vi "Save Data（Feedback）.vi"(6 "index":i32, 7 "Data":variant, 8 "error in (no error)":errorcluster caption="错误输入（无错误）", 9 "Code":string, 10 "Table":string, 11 "Connncet State":T1) -> (0 "error out":errorcluster caption="错误输出", 2 "State":bool)   [LabVIEW 2014]
uses:
  <vilib>/addons/database/NI_Database_API.lvlib
  Ctr/Constr.ctl
  <vilib>/addons/database/Connection.llb/Conn ObjectReference.ctl
  Ctr/Conneect State.ctl
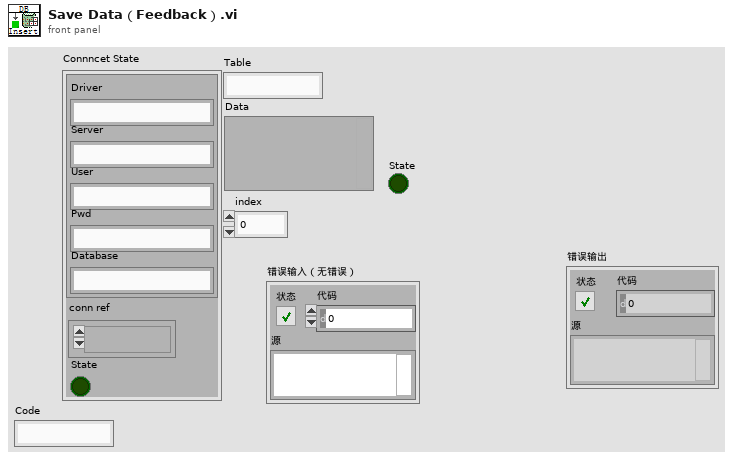
[diagram p1: front panel]
types:
  T1 = typedef "Conneect State.ctl" = cluster{"Constr":T2, "conn ref":T3, "State":bool}
  T2 = typedef "Constr.ctl" = cluster{"Driver":string, "Server":string, "User":string, "Pwd":string, "Database":string}
  T3 = typedef "NI_Database_API.lvlib/Conn ObjectReference.ctl" = refnum<k1>
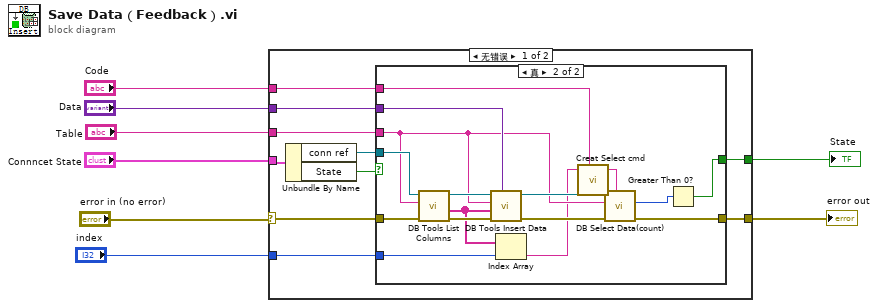
[diagram p0: block diagram]
diagram:
  n1 = case shown="无错误" "error in (no error)" {
    selector: "error in (no error)" -> [w16 w36]
    tunnel: "Connncet State" -> [w18 _]
    tunnel: "Table" -> [w14 _]
    tunnel: "Data" -> [w13 _]
    tunnel: "index" -> [w12 _]
    tunnel: "Code" -> [w11 _]
    tunnel: [w10 w36] -> w2
    tunnel: [w9 _] -> w1
    frame No Error {
      n2 = Unbundle By Name(w18) -> ("conn ref"=w15:T3, "State"=w17:bool)
      n3 = case shown="真" w17 {
        tunnel: w16 -> [w19 w35]
        tunnel: w15 -> [_ w34]
        tunnel: w14 -> [_ w26]
        tunnel: w13 -> [_ w31]
        tunnel: w12 -> [_ w29]
        tunnel: w11 -> [_ w24]
        tunnel: [w19 w23] -> w10
        tunnel: [_ w21] -> w9
        frame False {
        }
        frame True {
          n4 = call <vilib>:"DB Tools List Columns.vi"("error in (no error)"=w35, "table"=w26, "connection reference"=w34) -> ("error out"=w33:errorcluster, "columns"=w30:string[], "connection reference out"=w32:T3)  [unwired: 1 in, 1 out]
          n5 = call <vilib>:"DB Tools Insert Data.vi"("data"=w31, "error in (no error)"=w33, "columns"=w30, "table"=w26, "connection reference"=w32) -> ("error out"=w28:errorcluster, "connection reference out"=w27:T3)  [unwired: 5 in]
          n6 = Index Array(array=w30, index=w29) -> (element=w25:string)
          n7 = call "Creat Select cmd.vi"("Col"=w25, "Code"=w24) -> ("Str"=w20:string)  [unwired: 7 in]
          n8 = call "DB Select Data(count).vi"("condition"=w20, "error in (no error)"=w28, "table"=w26, "connection reference"=w27) -> ("error out"=w23:errorcluster, "Count"=w22:i32)  [unwired: 5 in, 1 out]
          n9 = Greater Than 0?(x=w22) -> (x > 0?=w21:bool)
        }
      }
    }
    frame Error {
    }
  }
  "error out" <- w2
  "State" <- w1
